vi "ClassPanel_o.vi"(8 "error in (no error)":errorcluster caption="entrée d'erreur (pas d'erreur)", 11 "AndorSpectro.lvclass":refnum<class "AndorSpectro.lvclass">) -> (0 "error out":errorcluster caption="sortie d'erreur", 3 "AndorSpectro.lvclass Out":refnum<class "AndorSpectro.lvclass">)   [LabVIEW 2019, in "AndorSpectro.lvclass"]
uses:
  AndorSpectro.lvclass
  C:/Programmes Labview/LabscanV1A/DevicesClass/BaseDevice/BaseDevice.lvclass
  <userlib>/ATSpectrograph/GUI/AndorNoiseCorr.ctl
  <userlib>/atmcd32d.llb/AndorCapabilities typedef.ctl
  <userlib>/atmcd32d.llb/TriggerMode_mode typedef.ctl
  <userlib>/atmcd32d.llb/AcquisitionMode_mode typedef.ctl
  <userlib>/atmcd32d.llb/ReadMode_mode typedef.ctl
  BaseDevice/ClassQueueMess.ctl
  AndorSpectro.lvclass/AndorSpectro.ctl
  BaseDevice/Accessor/GetClassEvent.vi
  <userlib>/ATSpectrograph/atspectrograph.lvlib
panel:
  out "Background":i32[](array[numeric])
  out "AndorMainQ":refnum<queue>
  out "Wavelength":sgl
  out "CalValues":sgl[](array[numeric])
  out "Detector offset":i32
  out "grating out":i32
  out "Grating offset":i32
  out "gain":sgl format="%.2f"
  out "information":i32
  out "caps":T1
  in  "X Start":i32=1 min=1 max=1023 step=1
  in  "X End":i32=1024 min=2 max=1024 step=1
  in  "Graph Number":i32 min=0 max=256 step=1
  in  "AndorTabs":enum32{"Main Controls", "Settings", "Data"}(tab)
  in  "AccDone":u16 caption="Acq. Done"
  in  "Stop Acq":bool
  in  "Con/Disc.":bool
  in  "Gain":i32(ring) caption="Device Name" items=["Gain  1.0(x)", "Gain  1.7(x)"]
  in  "Image Mode":bool=TRUE
  in  "AquireImage":bool caption="MiseAJour"
  out "AcqTime":sgl caption="Acq. Time (s)" format="%#.3f"
  in  "IntegTime":u32=100 caption="Integration\nTime (ms)" min=1 max=100000 step=1
  in  "Accumulation":u16=1 min=1 max=256 step=1
  out "Temp °C":i32
  in  "Cooler":bool
  in  "Save Data":bool caption="Save\nData"
  in  "Cont. Acq.":bool caption="Cont.\nAcq."
  out "Stable":bool
  in  "Setp. °C":i32=-80
  out "Aquiring":bool
  in  "Save Bckgnd":bool caption="Save as \nBckgnd"
  out "accumulate":sgl format="%.2f"
  in  "SetAreas":bool caption="MiseAJour"
  in  "Y Bins":i32=1 min=1 max=256 step=1
  out "areas":i32[][](array[numeric])=[[1], [1], [1], [1024], [256], [1], [256]]
  in  "HS":u16(ring) caption="Hor. Spd." items=["33kHz@16bit", "50kHz@16bit", "100kHz@16bit"]
  in  "VS":u16(ring)=1 caption="Vert. Spd (us)" items=["[8.25]", "16.25", "32.25", "64.25"]
  in  "Y End":i32=256 min=2 max=256 step=1
  in  "Y Start":i32=1 min=1 max=255 step=1
  in  "Backgnd Mode":T2=enum."Selected Curve"
  in  "NoiseWindow":bool caption="Noise Window"
  out "Cosmic Filter":bool
  in  "MainProgQ":refnum<queue>
  in  "MainProgQEvent":refnum<user-event>
  in  "Acq":bool
  in  "Stop":bool
  out "Init Program":bool
  # "Andor Camera"
  # "this MUST labeled with class name"
  # "this MUST be present and labeled \"Stop\" and \"Acq\""
  # "Single Acq"
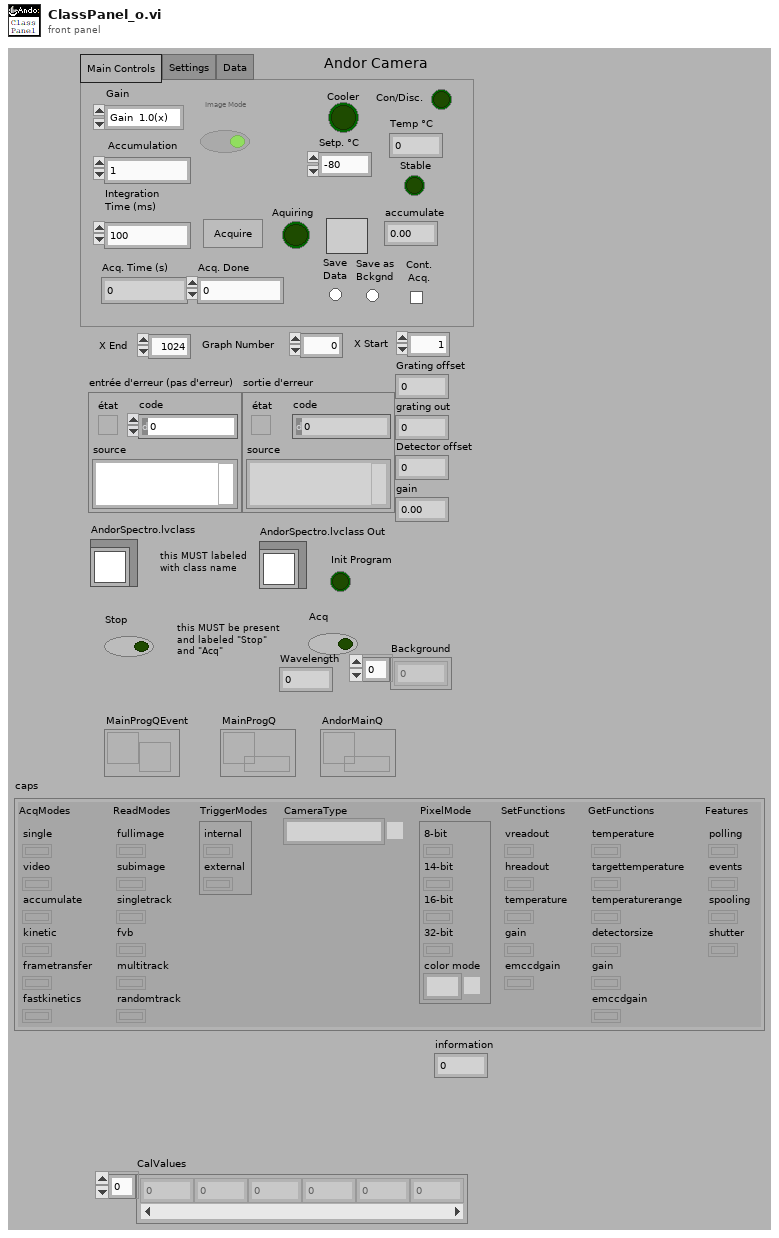
[diagram p1: front panel]
types:
  T1 = typedef "AndorCapabilities typedef.ctl" = cluster{"AcqModes":cluster{"single":bool, "video":bool, "accumulate":bool, "kinetic":bool, "frametransfer":bool, "fastkinetics":bool}, "ReadModes":cluster{"fullimage":bool, "subimage":bool, "singletrack":bool, "fvb":bool, "multitrack":bool, "randomtrack":bool}, "TriggerModes":cluster{"internal":bool, "external":bool}, "CameraType":enum32{"PDA", "iXon", "ICCD", "EMCCD", "CCD", "iStar", "third party camera", "iDus", "Newton", "Surcam", "USB ICCD", "Luca", "Reserved", "iKon", "InGaAs", "iVac", "Unprogrammed", "Clara", "USB iStar", "SimCam", "Neo", "iXon Ultra", "Volmos", "iVac Ultra"}, "PixelMode":cluster{"8-bit":bool, "14-bit":bool, "16-bit":bool, "32-bit":bool, "color mode":enum16{"Mono", "RGB", "CMY"}}, "SetFunctions":cluster{"vreadout":bool, "hreadout":bool, "temperature":bool, "gain":bool, "emccdgain":bool}, "GetFunctions":cluster{"temperature":bool, "targettemperature":bool, "temperaturerange":bool, "detectorsize":bool, "gain":bool, "emccdgain":bool}, "Features":cluster{"polling":bool, "events":bool, "spooling":bool, "shutter":bool}}
  T2 = typedef "AndorNoiseCorr.ctl" = enum16{"Off", "Selected Curve", "One For Every Acq"}
  T3 = cluster{"Message":string, "Data":variant, "Code":i32}
  T4 = typedef "ReadMode_mode typedef.ctl" = enum16{"Full Vertical Binning", "Multi-Track", "Random-Track", "Single-Track", "Image"}
  T5 = typedef "AcquisitionMode_mode typedef.ctl" = enum16{"Reserved (0)", "Single Scan", "Accumulate", "Kinetics", "Fast Kinetics", "Run Till Abort", "Reserved (6)", "Reserved (7)", "Reserved (8)", "Time Delayed Integration"}
  T6 = typedef "TriggerMode_mode typedef.ctl" = enum16{"Internal", "External", "N/A (2)", "N/A (3)", "N/A (4)", "N/A (5)", "External Start"}
  T7 = typedef "ClassQueueMess.ctl" = u16
  T8 = cluster{"wavelength out":sgl, "calibrationValuesOut":sgl[], "gain":sgl, bool}
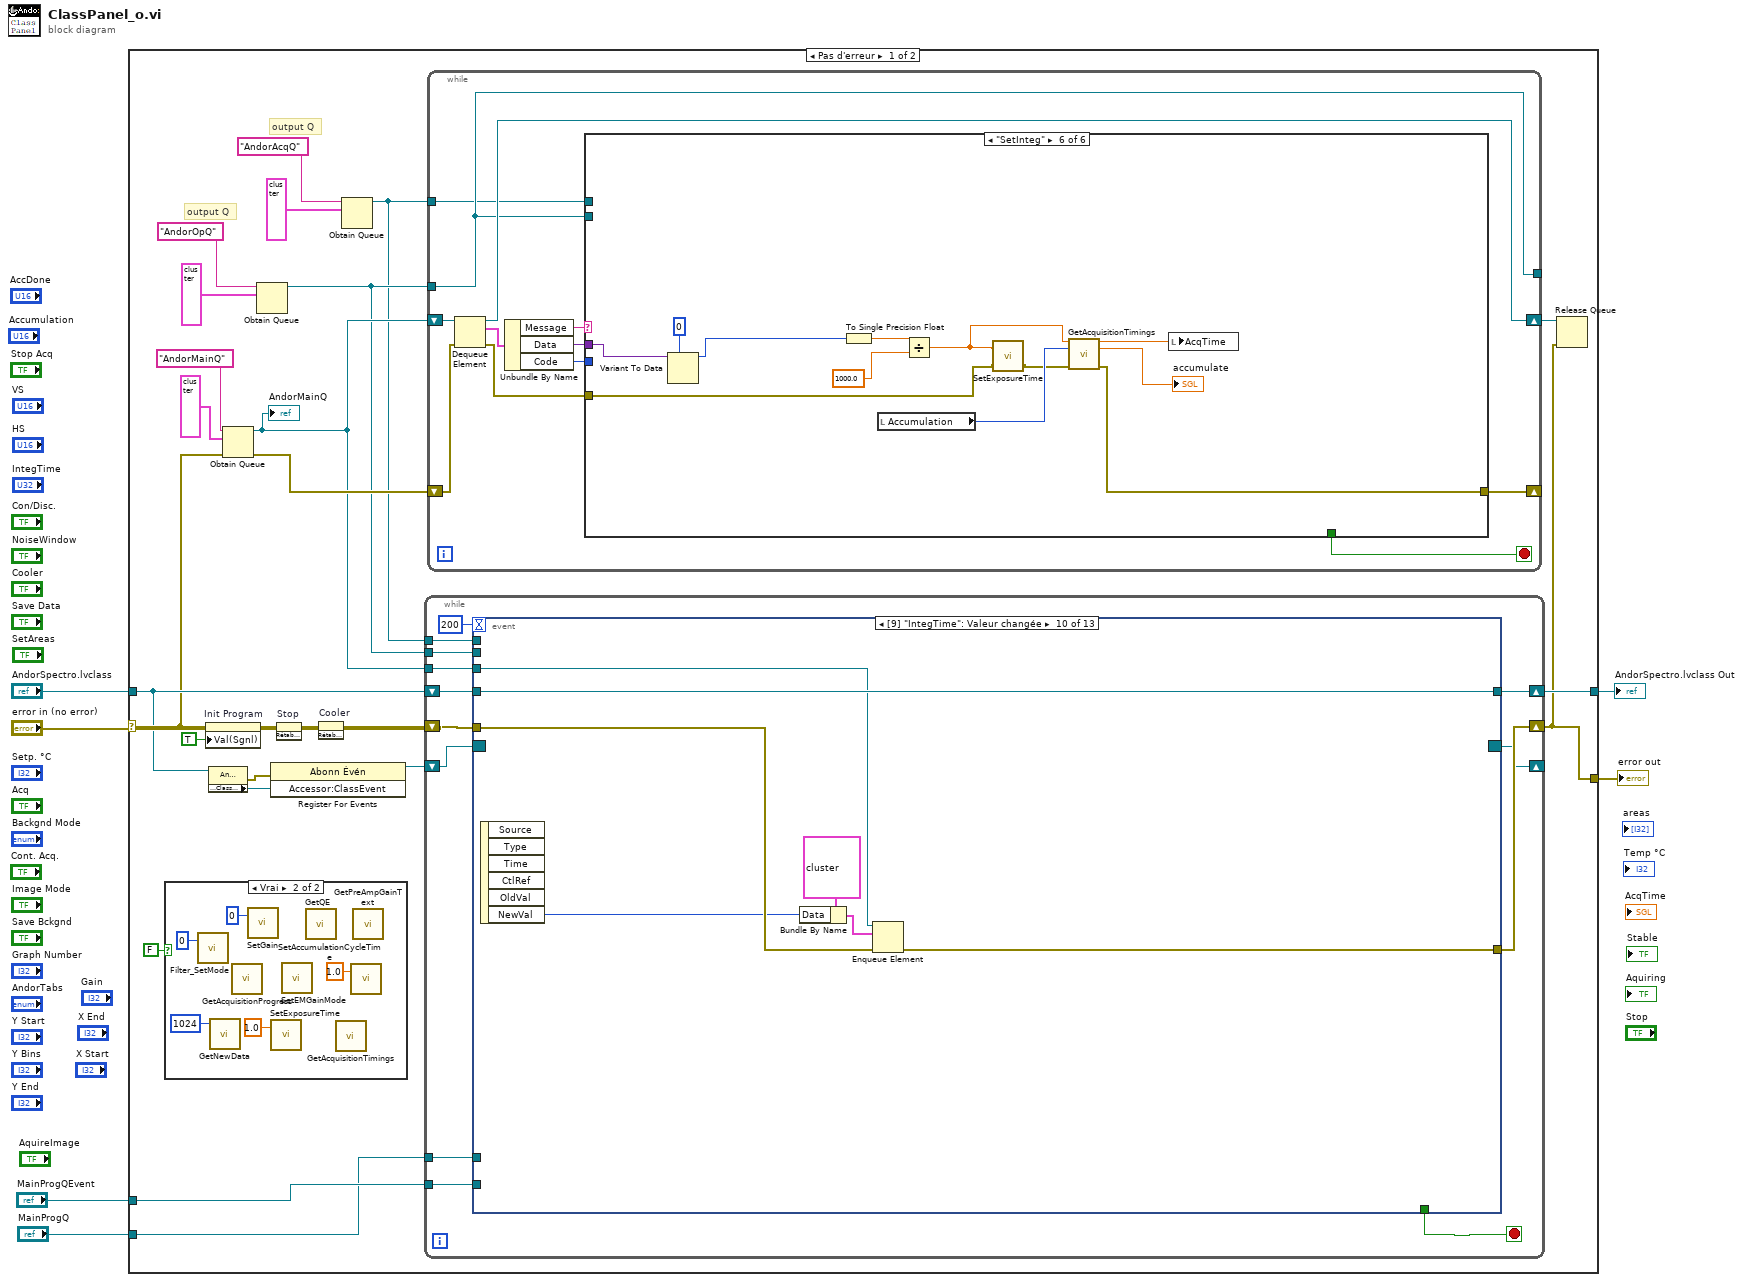
[diagram p0: block diagram]
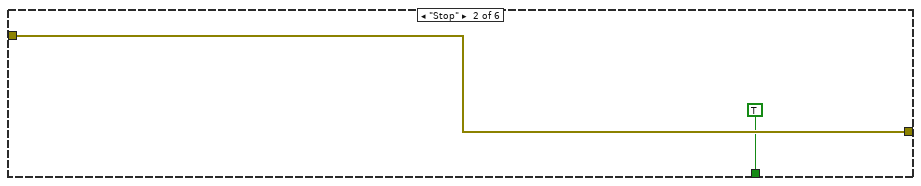
[diagram p4: hidden frame]
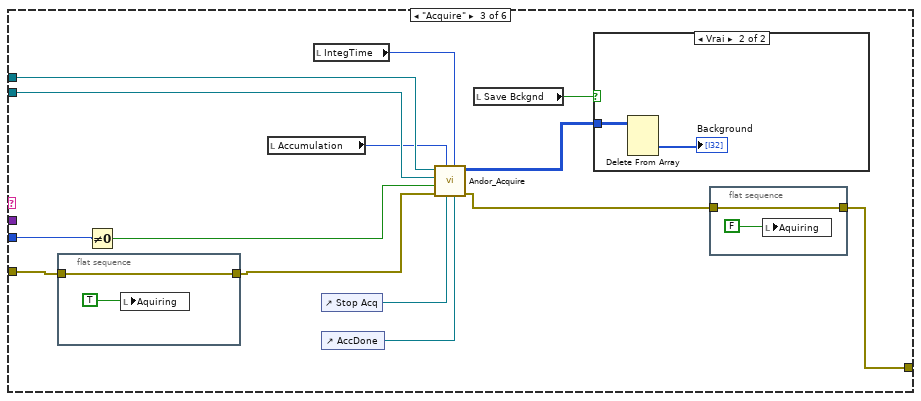
[diagram p5: hidden frame]
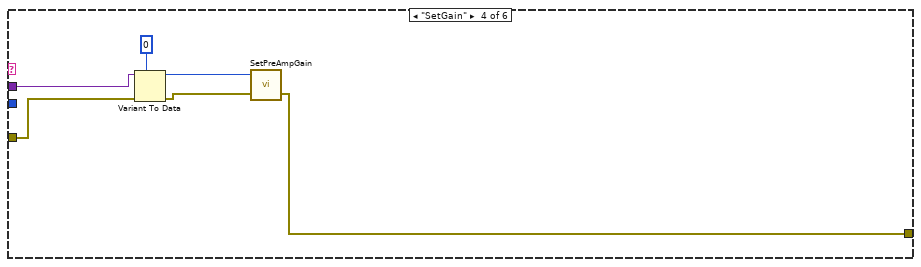
[diagram p7: hidden frame]
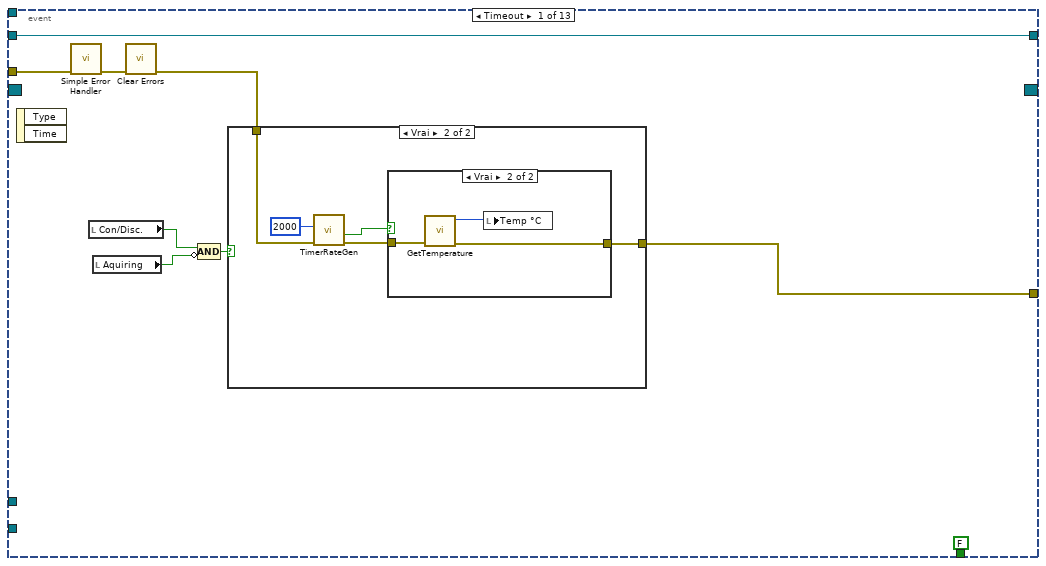
[diagram p9: hidden frame]
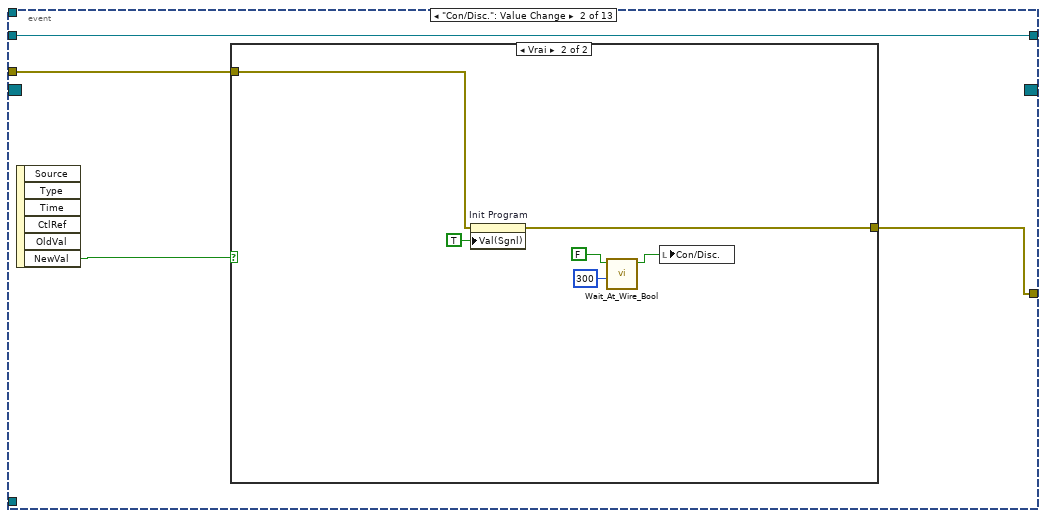
[diagram p12: hidden frame]
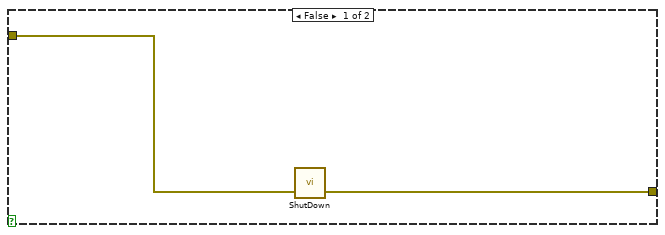
[diagram p13: hidden frame]
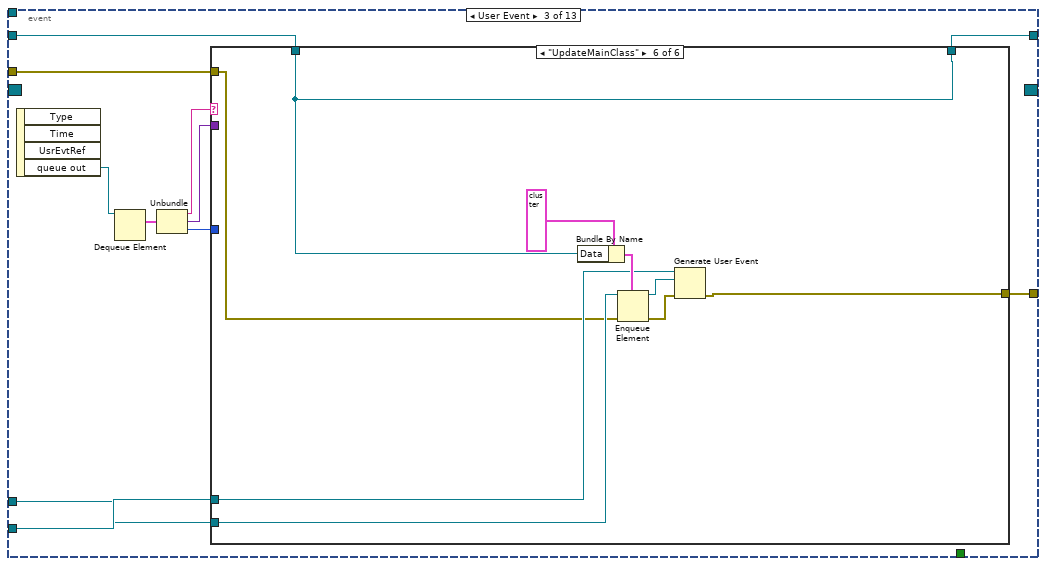
[diagram p14: hidden frame]
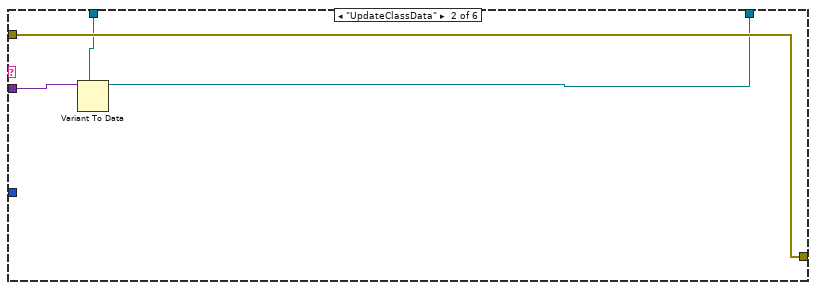
[diagram p16: hidden frame]
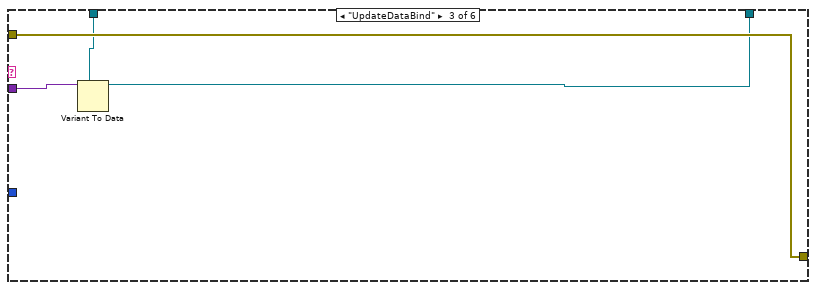
[diagram p17: hidden frame]
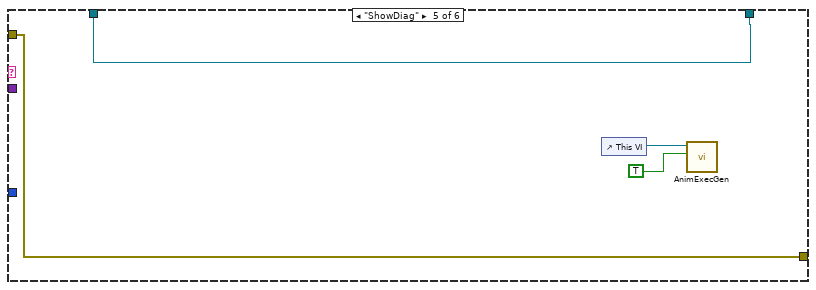
[diagram p19: hidden frame]
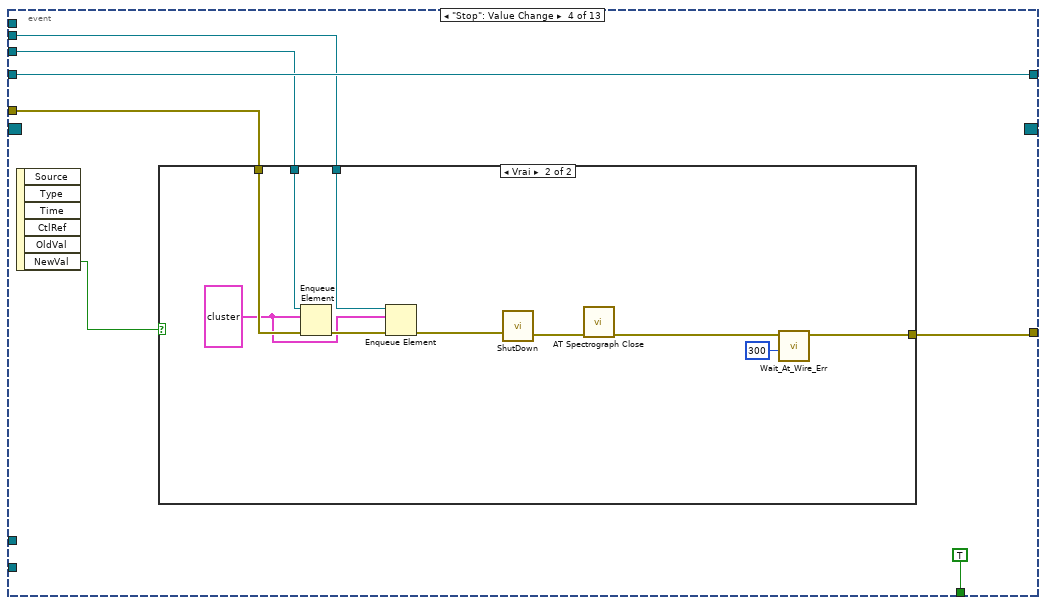
[diagram p20: hidden frame]
diagram:
  n1 = case shown="Pas d'erreur" "error in (no error)" {
    selector: "error in (no error)" -> [w21 w397]
    tunnel: [w7 w397] -> w5
    tunnel: "AndorSpectro.lvclass" -> [w26 w396]
    tunnel: [w30 w396] -> w3
    tunnel: "MainProgQEvent" -> [w24 _]
    tunnel: "MainProgQ" -> [w23 _]
    frame No Error {
      # "output Q"
      # "output Q"
      n2 = case shown="Vrai" FALSE {
        frame False {
        }
        frame True {
          n3 = call <userlib>:"Filter_SetMode.vi"("Mode"=u32 0) -> ()  [unwired: 1 in, 2 out]
          n4 = call <userlib>:"GetNewData.vi"("size"=u32 1024) -> ()  [unwired: 2 in, 3 out]
          n5 = call <userlib>:"GetAcquisitionProgress.vi"() -> ()  [unwired: 4 in, 4 out]
          n6 = call <userlib>:"SetGain.vi"("gain"=0) -> ()  [unwired: 1 in, 2 out]
          n7 = call <userlib>:"SetExposureTime.vi"("time"=sgl 1.0) -> ()  [unwired: 1 in, 2 out]
          n8 = call <userlib>:"SetEMGainMode.vi"() -> ()  [unwired: 2 in, 2 out]
          n9 = call <userlib>:"GetQE.vi"() -> ()  [unwired: 4 in, 3 out]
          n10 = call <userlib>:"GetAcquisitionTimings.vi"() -> ()  [unwired: 11 in, 5 out]
          n11 = call <userlib>:"SetAccumulationCycleTime.vi"("time"=sgl 1.0) -> ()  [unwired: 1 in, 2 out]
          n12 = call <userlib>:"GetPreAmpGainText.vi"() -> ()  [unwired: 2 in, 3 out]
        }
      }
      n13 = property on="Init Program" class="Bool (strict)"(error in=w21, "Val(Sgnl)"=TRUE ("Valeur (Signalisation)")) -> (error out=w29:errorcluster)  [unwired: 1 in, 1 out]
      n14 = property class="AndorSpectro.lvclass"(reference=w26) -> (error out=w28:errorcluster, "Accessor:ClassEvent"=w27:refnum<user-event>)  [unwired: 1 in, 1 out]
      n15 = Obtain Queue(name (unnamed)="AndorMainQ" ("nom (aucun)"), element data type=T3 {"Message"="", "Data"=variant, "Code"=0}, error in (no error)=w21) -> (queue out=w18:refnum<queue>, error out=w20:errorcluster)  [unwired: 2 in, 1 out]
      "AndorMainQ" <- w18
      n16 = Obtain Queue(name (unnamed)="AndorOpQ" ("nom (aucun)"), element data type=T3 {"Message"="", "Data"=variant, "Code"=0} ("element")) -> (queue out=w11:refnum<queue>)  [unwired: 3 in, 2 out]
      n17 = register-events(error in=w28, w27) -> (reference out=w25:refnum<event-registration>)  [unwired: 1 in, 1 out]
      n18 = invoke on="Stop" class="Bool (strict)" method="RétablirValParDéfaut"(error in=w29) -> (error out=w13:errorcluster)  [unwired: 2 in, 2 out]
      n19 = invoke on="Cooler" class="Bool (strict)" method="RétablirValParDéfaut"(error in=w13) -> (error out=w12:errorcluster)  [unwired: 2 in, 2 out]
      n20 = Obtain Queue(name (unnamed)="AndorAcqQ" ("nom (aucun)"), element data type=T3 {"Message"="", "Data"=variant, "Code"=0} ("element")) -> (queue out=w8:refnum<queue>)  [unwired: 3 in, 2 out]
      n21 = while {
        shift-right: [w101] -> w7
        shift-left: w12 -> [w102]
        shift-right: [w99] -> w30
        shift-left: w26 -> [w100]
        shift-right: [w97] -> _
        shift-left: w25 -> [w98]
        tunnel: w24 -> [w96]
        tunnel: w23 -> [w95]
        tunnel: w18 -> [w94]
        tunnel: w11 -> [w93]
        tunnel: w8 -> [w92]
        stop <- w91 stop-if-true
        n22 = event shown="[9] \"IntegTime\": Valeur changée" {
          selector: w98 -> [_ _ _ _ _ _ _ _ _ _ _ _ _]
          dyn-events: [_ _ _ _ _ _ _ _ _ _ _ _ _] -> w97
          timeout: 200 -> [_ _ _ _ _ _ _ _ _ _ _ _ _]
          tunnel: w102 -> [w110 w125 w144 w174 w189 w197 w293 w305 w315 w325 w335 w372 w391]
          tunnel: [w106 w123 w138 w172 w189 w199 w289 w304 w314 w327 w331 w371 w390] -> w101
          tunnel: w100 -> [w111 w124 w145 w176 w190 w194 w294 w306 w317 w328 w336 w373 w395]
          tunnel: [FALSE _ _ TRUE _ FALSE _ _ _ _ _ _ _] -> w91
          tunnel: [w111 w124 w137 w176 w190 w193 w294 w306 w317 w328 w332 w373 w395] -> w99
          tunnel: w96 -> [_ _ w136 _ _ _ _ _ _ _ w333 _ _]
          tunnel: w95 -> [_ _ w135 _ _ _ _ _ _ _ w334 _ _]
          tunnel: w94 -> [_ _ _ w175 _ w195 w288 _ _ w326 w330 _ w389]
          tunnel: w93 -> [_ _ _ w173 _ w196 _ _ _ _ w329 _ _]
          tunnel: w92 -> [_ _ _ _ _ w192 _ _ _ _ _ _ _]
          event Timeout {
            n23 = event-data() -> ()  [unwired: 1 in, 2 out]
            n24 = call <vilib>:"Simple Error Handler.vi"("error in (no error)"=w110) -> ("error out"=w109:errorcluster)  [unwired: 4 in, 4 out]
            n25 = local read "Con/Disc."() -> (w108:bool)
            n26 = local read "Aquiring"() -> (w104:bool)
            n27 = call <vilib>:"Clear Errors.vi"("error in (no error)"=w109) -> ("error out"=w107:errorcluster)  [unwired: 5 in, 1 out]
            n28 = Compound Arithmetic op=AND ("Opérateur arithmétique")(w108, invert w104) -> (w105:bool)
            n29 = case shown="Vrai" w105 {
              tunnel: w107 -> [w113 w117]
              tunnel: [w113 w115] -> w106
              frame False {
              }
              frame True {
                n30 = call <userlib>:"TimerRateGen.vi"("error in (no error)"=w117, "Refresh(ms)"=u32 2000) -> ("error out"=w116:errorcluster, "updated?"=w114:bool)  [unwired: 7 in, 1 out]
                n31 = case shown="Vrai" w114 {
                  tunnel: w116 -> [w119 w122]
                  tunnel: [w119 w120] -> w115
                  frame False {
                  }
                  frame True {
                    n32 = call <userlib>:"GetTemperature.vi"("error in (no error)"=w122) -> ("error out"=w120:errorcluster, "temperature"=w121:i32)  [unwired: 3 in, 2 out]
                    n33 = local write "Temp °C"(w121) -> ()
                  }
                }
              }
            }
          }
          event "Con/Disc.": Value Change {
            n34 = event-data() -> ("NewVal"=w126:bool)  [unwired: 1 in, 5 out]
            n35 = case shown="Vrai" w126 {
              tunnel: w125 -> [w128 w133]
              tunnel: [w127 w132] -> w123
              frame False {
                n36 = call <userlib>:"ShutDown.vi"("error in (no error)"=w128) -> ("error out"=w127:errorcluster)  [unwired: 1 in, 1 out]
              }
              frame True {
                n37 = property on="Init Program" class="Bool (strict)"(error in=w133, "Val(Sgnl)"=TRUE ("Valeur (Signalisation)")) -> (error out=w132:errorcluster)  [unwired: 1 in, 1 out]
                n38 = call <userlib>:"Wait_At_Wire_Bool.vi"("Wait (ms)"=u32 300, "error in (no error)"=FALSE ("Con/Disc.")) -> ("error out"=w130:bool)  [unwired: 7 in, 2 out]
                n39 = local write "Con/Disc."(w130) -> ()
              }
            }
          }
          event User Event {
            n40 = event-data() -> ("queue out"=w142:refnum<queue>)  [unwired: 1 in, 3 out]
            n41 = Dequeue Element(queue=w142) -> (element=w143:cluster{"Message":string, "Data":variant, i32})  [unwired: 2 in, 3 out]
            n42 = Unbundle(w143) -> ("Message"=w141:string, "Data"=w140:variant, w139:i32)
            n43 = case shown="\"UpdateMainClass\"" w141 {
              tunnel: w144 -> [w147 w151 w155 w156 w160 w163]
              tunnel: w140 -> [_ w150 w154 _ _ _]
              tunnel: w145 -> [w146 w149 w153 w157 w161 w166]
              tunnel: [w146 w148 w152 w157 w161 w166] -> w137
              tunnel: [w147 w151 w155 w156 w160 w162] -> w138
              tunnel: w139 -> [_ _ _ _ _ _]
              tunnel: w136 -> [_ _ _ _ _ w165]
              tunnel: w135 -> [_ _ _ _ _ w164]
              frame Default {
              }
              frame "UpdateClassData" {
                n44 = Variant To Data(type=w149, Variant=w150) -> (data=w148:refnum<class "AndorSpectro.lvclass">)  [unwired: 1 in, 1 out]
              }
              frame "UpdateDataBind" {
                n45 = Variant To Data(type=w153, Variant=w154) -> (data=w152:refnum<class "AndorSpectro.lvclass">)  [unwired: 1 in, 1 out]
              }
              frame "MeasDone" {
              }
              frame "ShowDiag" {
                n46 = control-ref of="This VI"() -> (w159:refnum<vi>)
                n47 = call <userlib>:"AnimExecGen.vi"("Animer l'exécution ?"=TRUE, "ViRef"=w159) -> ()  [unwired: 9 in, 1 out]
              }
              frame "UpdateMainClass" {
                n48 = Bundle By Name(cluster=cluster{"Message":string, "Data":variant, i32} {"Message"="", "Data"=variant, 0} ("élément"), "Data"=w166) -> (w167:cluster{"Message":string, "Data":variant, i32})
                n49 = Enqueue Element(queue=w164, element=w167, error in (no error)=w163) -> (queue out=w170:refnum<queue>, error out=w169:errorcluster)  [unwired: 1 in, 1 out]
                n50 = Generate User Event(user event=w165, event data cluster=w170, error in=w169) -> (error out=w162:errorcluster)  [unwired: 1 in, 1 out]
              }
            }
          }
          event "Stop": Value Change {
            n51 = event-data() -> ("NewVal"=w171:bool)  [unwired: 1 in, 5 out]
            n52 = case shown="Vrai" w171 {
              tunnel: w175 -> [_ w188]
              tunnel: w174 -> [w178 w187]
              tunnel: w173 -> [_ w183]
              tunnel: [w178 w180] -> w172
              frame False {
              }
              frame True {
                w182 = T3 {"Message"="Stop", "Data"=variant, "Code"=0} ("élément")
                n53 = Enqueue Element(queue=w188, element=w182, error in (no error)=w187) -> (error out=w184:errorcluster)  [unwired: 1 in, 2 out]
                n54 = Enqueue Element(queue=w183, element=w182, error in (no error)=w184) -> (error out=w181:errorcluster)  [unwired: 1 in, 2 out]
                n55 = call <userlib>:"ShutDown.vi"("error in (no error)"=w181) -> ("error out"=w186:errorcluster)  [unwired: 1 in, 1 out]
                n56 = call <userlib>:"AT Spectrograph Close.vi"("error in (no error)"=w186) -> ("error out"=w185:errorcluster)  [unwired: 9 in, 1 out]
                n57 = call <userlib>:"Wait_At_Wire_Err.vi"("Wait (ms)"=u32 300, "error in (no error)"=w185) -> ("error out"=w180:errorcluster)  [unwired: 7 in, 2 out]
              }
            }
          }
          event Panel Close? {
            n58 = event-data() -> ()  [unwired: 1 in, 4 out]
            n59 = event-data("Discard?"=TRUE ("Rejeter ?")) -> ()  [unwired: 1 in, 1 out]
          }
          event "Init Program": Value Change {
            n60 = event-data() -> ("NewVal"=w200:bool)  [unwired: 1 in, 4 out]
            n61 = case shown="Vrai" w200 {
              tunnel: w197 -> [w202 w204]
              tunnel: [w202 w222] -> w199
              tunnel: [_ w240] -> _
              tunnel: [_ w239] -> _
              tunnel: [_ w235] -> _
              tunnel: [_ w221] -> _
              tunnel: w196 -> [_ w215]
              tunnel: w195 -> [_ w209]
              tunnel: w194 -> [w201 w216]
              tunnel: [w201 w211] -> w193
              tunnel: w192 -> [_ w210]
              frame False {
              }
              frame True {
                w213 = T7 1 items=["UpdateClassData", "UpdateMainClass", "UpdateDataBind", "ReInitDevice", "Custom", "ClosePan"] ("Menu déroulant")
                w245 = u32 0 items=["DIRECT", "SIDE"] ("entrancePort")
                w246 = u32 0 items=["DIRECT", "SIDE"] ("exitPort")
                w229 = 0
                w231 = 0
                w254 = 0 ("index")
                w274 = -80 ("temperature")
                w271 = 0
                w283 = u32 20002  # DRV_SUCCESS
                n62 = call <userlib>:"Initialize.vi"("error in (no error)"=w204, "directory (\"\")"="" ("directory (\"\")")) -> ("error out"=w264:errorcluster, "DLL error code"=w284:u32)
                n63 = local write "Image Mode"(FALSE ("Image Mode")) -> ()
                n64 = call <userlib>:"Wait_At_Wire_Err.vi"("Wait (ms)"=u32 2000, "error in (no error)"=w264) -> ("error out"=w262:errorcluster)  [unwired: 7 in, 2 out]
                n65 = Equal?(x=w284, y=w283) -> (x = y?=w260:bool)
                n66 = Open VI Reference(type specifier VI Refnum (for type only)=refnum<vi> refnum ("référence"), vi path=path "C:/Program Files (x86)/National Instruments/LabVIEW 2019/user.lib/ATSpectrograph/GUI/Andor_Operate.vi" ("chemin du VI"), options=128, error in (no error)=w204) -> (vi reference=w205:refnum<vi>, error out=w203:errorcluster)  [unwired: 2 in]
                n67 = call <userlib>:"GetCameraInformation.vi"("error in (no error)"=w262) -> ("error out"=w263:errorcluster, "information"=w259:i32)  [unwired: 2 in, 1 out]
                "information" <- w259
                n68 = Equal?(x=7, y=w259) -> (x = y?=w257:bool)
                n69 = call-by-ref "Démarrer un appel asynchrone"(reference=w205, error in=w203, 8:"error in (no error)"=w204, "AndorAcqQ"=w209, "AndorOpQ"=w215) -> ()  [unwired: 8 in, 3 out]
                n70 = call <userlib>:"GetCapabilities.vi"("error in (no error)"=w263) -> ("error out"=w261:errorcluster, "caps"=→"caps":T1)  [unwired: 2 in, 1 out]
                n71 = And(x=w260, y=w257) -> (x .and. y?=w217:bool)
                n72 = local write "Con/Disc."(w217) -> ()
                n73 = property on="Accumulation" class="NumNb (strict)"("Value"=u16 1 ("Accumulation")) -> ()  [unwired: 2 in, 2 out]
                n74 = call <userlib>:"SetReadMode.vi"("error in (no error)"=w261, "mode"=ReadMode_mode_typedef."Full Vertical Binning") -> ("error out"=w280:errorcluster)  [unwired: 1 out]
                n75 = call <userlib>:"SetAcquisitionMode.vi"("error in (no error)"=w280, "mode"=AcquisitionMode_mode_typedef."Single Scan") -> ("error out"=w253:errorcluster)  [unwired: 1 out]
                n76 = local write "Setp. °C"(w274) -> ()
                n77 = Bundle By Name(cluster=w216, "AndorOpQ"=w215, "AndorAcqQ"=w210, "AndorMainQ"=w209) -> (w214:refnum<class "AndorSpectro.lvclass">)
                n78 = call <userlib>:"GetPreAmpGain.vi"("error in (no error)"=w253, "index"=w254) -> ("gain"=w218:sgl)  [unwired: 1 in, 2 out]
                "gain" <- w218
                n79 = call <userlib>:"SetPreAmpGain.vi"("error in (no error)"=w253, "index"=w254) -> ("error out"=w268:errorcluster)  [unwired: 1 out]
                n80 = property on="Gain" class="MDér (strict)"(error in=w253, "Value"=w254) -> (error out=w267:errorcluster)  [unwired: 1 in, 1 out]
                n81 = call <userlib>:"SetHSSpeed.vi"("error in (no error)"=w268, "index"=w271, "type"=w271) -> ("error out"=w277:errorcluster)  [unwired: 1 in, 1 out]
                n82 = property on="HS" class="MDér (strict)"(error in=w267, "Value"=w271) -> (error out=w266:errorcluster)  [unwired: 1 in, 1 out]
                n83 = call <userlib>:"GetNumberVSSpeeds.vi"("error in (no error)"=w277) -> ("error out"=w276:errorcluster, "number"=w278:i32)  [unwired: 2 in, 1 out]
                n84 = Subtract(x=w278, y=1) -> (x-y=w272:i32)
                n85 = call <userlib>:"SetVSSpeed.vi"("error in (no error)"=w276, "index"=w272) -> ("error out"=w241:errorcluster)  [unwired: 1 out]
                n86 = property on="VS" class="MDér (strict)"(error in=w266, "Value"=w272) -> (error out=w212:errorcluster)  [unwired: 1 in, 1 out]
                n87 = call <userlib>:"GetPixelSize.vi"("error in (no error)"=w241) -> ("error out"=w242:errorcluster, "ysize"=w239:sgl, "xsize"=w240:sgl)  [unwired: 3 in, 1 out]
                n88 = call-dynamic "SetClassQueueMessage.vi"("ErrorIn(No Error)"=w212, "Menu déroulant"=w213, "DefaultDev.lvclass"=w214) -> ("DefaultDev.lvclass Out"=w211:refnum<class "AndorSpectro.lvclass">)  [unwired: 7 in, 1 out]
                n89 = call <userlib>:"GetFilterMode.vi"("error in (no error)"=w242) -> ("error out"=w238:errorcluster, "mode"=→"Cosmic Filter":bool)  [unwired: 2 in, 1 out]
                n90 = call <userlib>:"SetTemperature.vi"("error in (no error)"=w238, "temperature"=w274) -> ("error out"=w273:errorcluster)  [unwired: 1 out]
                n91 = call <userlib>:"SetTriggerMode.vi"("error in (no error)"=w273, "mode"=TriggerMode_mode_typedef."Internal") -> ("error out"=w234:errorcluster)  [unwired: 1 out]
                n92 = property on="IntegTime" class="NumNb (strict)"(error in=w234, "Val(Sgnl)"=u32 100 ("Valeur (Signalisation)")) -> (error out=w237:errorcluster)  [unwired: 1 in, 1 out]
                n93 = call <userlib>:"AT Spectrograph Initialize.vi"("error in (no error)"=w237, "iniPath"="") -> ("error out"=w233:errorcluster, "function return"=w235:u32)  [unwired: 8 in]
                n94 = call <userlib>:"AT Spectrograph Get Wavelength.vi"("error in (no error)"=w233, "device"=w231) -> ("error out"=w232:errorcluster, "wavelength out"=w221:sgl)  [unwired: 7 in, 1 out]
                "Wavelength" <- w221
                n95 = call <userlib>:"AT Spectrograph Set Pixel Width.vi"("error in (no error)"=w232, "width"=sgl 26.0, "device"=w231) -> ("error out"=w251:errorcluster)  [unwired: 7 in, 1 out]
                n96 = call <userlib>:"AT Spectrograph Set Number Pixels.vi"("error in (no error)"=w251, "numberPixels"=1024, "device"=w231) -> ("error out"=w227:errorcluster)  [unwired: 7 in, 1 out]
                n97 = call <userlib>:"AT Spectrograph Get Grating.vi"("error in (no error)"=w227, "device"=w229) -> ("error out"=w226:errorcluster, "grating out"=w247:i32)  [unwired: 7 in, 1 out]
                "grating out" <- w247
                n98 = call <userlib>:"AT Spectrograph Get Grating Offset.vi"("error in (no error)"=w226, "grating"=w247, "device"=w229) -> ("error out"=w249:errorcluster, "offset out"=→"Grating offset":i32)  [unwired: 6 in, 1 out]
                n99 = call <userlib>:"AT Spectrograph Get Detector Offset.vi"("error in (no error)"=w249, "exitPort"=w246, "entrancePort"=w245, "device"=w229) -> ("error out"=w228:errorcluster, "offset out"=→"Detector offset":i32)  [unwired: 5 in, 1 out]
                n100 = call <userlib>:"AT Spectrograph Get Calibration.vi"("error in (no error)"=w228, "numberPixels"=1024, "device"=w229) -> ("error out"=w223:errorcluster, "calibrationValuesOut"=w220:sgl[])  [unwired: 5 in, 1 out]
                "CalValues" <- w220
                n101 = Bundle("wavelength out"=w221, "calibrationValuesOut"=w220, "gain"=w218, w217) -> (w219:T8)  [unwired: 1 in]
                n102 = Bundle By Name(cluster=T3 {"Message"="InitOp", "Data"=variant, "Code"=1}, "Data"=w219) -> (w225:T3)
                n103 = Enqueue Element(queue=w215, element=w225, error in (no error)=w223) -> (error out=w222:errorcluster)  [unwired: 1 in, 2 out]
                "Init Program" <- FALSE
              }
            }
          }
          event "Accumulation": Value Change {
            n104 = event-data() -> ("NewVal"=w295:u16)  [unwired: 1 in, 5 out]
            n105 = case shown="1" w295 {
              selector: w295 -> [w296 _]
              tunnel: w293 -> [w300 w303]
              tunnel: [w297 w302] -> w290
              frame Default {
                n106 = call <userlib>:"SetAcquisitionMode.vi"("error in (no error)"=w300, "mode"=AcquisitionMode_mode_typedef."Accumulate") -> ("error out"=w298:errorcluster)  [unwired: 1 out]
                n107 = call <userlib>:"SetNumberAccumulations.vi"("error in (no error)"=w298, "number"=w296) -> ("error out"=w297:errorcluster)  [unwired: 1 out]
              }
              frame 1 {
                # "Single scan mode"
                n108 = call <userlib>:"SetAcquisitionMode.vi"("error in (no error)"=w303, "mode"=AcquisitionMode_mode_typedef."Single Scan") -> ("error out"=w302:errorcluster)  [unwired: 1 out]
              }
            }
            n109 = local read "IntegTime"() -> (w287:u32)
            n110 = Bundle By Name(cluster=T3 {"Message"="SetInteg", "Data"=variant, "Code"=0}, "Data"=w287) -> (w291:T3)
            n111 = Enqueue Element(queue=w288, element=w291, error in (no error)=w290) -> (error out=w289:errorcluster)  [unwired: 1 in, 2 out]
          }
          event "Cont. Acq.": Value Change {
            n112 = event-data() -> ("NewVal"=w307:bool)  [unwired: 1 in, 5 out]
            n113 = case shown="Faux" w307 {
              tunnel: w305 -> [w310 w312]
              tunnel: [w309 w311] -> w304
              frame False {
                n114 = local read "Accumulation"() -> (w308:u16)
                n115 = property on="Accumulation" class="NumNb (strict)"(error in=w310, "Val(Sgnl)"=w308) -> (error out=w309:errorcluster)  [unwired: 1 in, 1 out]
              }
              frame True {
                n116 = call <userlib>:"SetAcquisitionMode.vi"("error in (no error)"=w312, "mode"=AcquisitionMode_mode_typedef."Run Till Abort") -> ("error out"=w311:errorcluster)  [unwired: 1 out]
              }
            }
          }
          event "Cooler": Value Change {
            n117 = event-data() -> ("NewVal"=w316:bool)  [unwired: 1 in, 5 out]
            n118 = case shown="Faux" w316 {
              tunnel: w315 -> [w319 w321]
              tunnel: [w318 w320] -> w314
              frame False {
                n119 = call <userlib>:"CoolerOFF.vi"("error in (no error)"=w319) -> ("error out"=w318:errorcluster)  [unwired: 1 in, 1 out]
              }
              frame True {
                n120 = call <userlib>:"CoolerON.vi"("error in (no error)"=w321) -> ("error out"=w320:errorcluster)  [unwired: 1 in, 1 out]
              }
            }
          }
          event "IntegTime": Value Change {
            n121 = event-data() -> ("NewVal"=w322:u32)  [unwired: 1 in, 5 out]
            n122 = Bundle By Name(cluster=T3 {"Message"="SetInteg", "Data"=variant, "Code"=0}, "Data"=w322) -> (w323:T3)
            n123 = Enqueue Element(queue=w326, element=w323, error in (no error)=w325) -> (error out=w327:errorcluster)  [unwired: 1 in, 2 out]
          }
          event "AquireImage": Value Change {
            n124 = event-data() -> ("NewVal"=w337:bool)  [unwired: 1 in]
            n125 = case shown="Vrai" w337 {
              tunnel: w336 -> [w338 w351]
              tunnel: w335 -> [w339 w342]
              tunnel: w334 -> [_ w349]
              tunnel: w333 -> [_ w350]
              tunnel: [w338 w348] -> w332
              tunnel: [w339 w346] -> w331
              tunnel: w330 -> [_ w340]
              tunnel: w329 -> [_ _]
              frame False {
              }
              frame True {
                n126 = local read "Save Data"() -> (w341:bool)
                n127 = property class="AndorSpectro.lvclass"(reference=w351, error in=w342) -> (reference out=w348:refnum<class "AndorSpectro.lvclass">, error out=w347:errorcluster, "Accessor:Function"=w356:string, "Accessor:InstrumentName"=w354:string)
                n128 = Concatenate Strings(w356, "@" ("chaîne"), w354) -> (w352:string)
                n129 = Bundle(w352, "Save Data"=w341) -> (w353:cluster{string, "Save Data":bool})  [unwired: 1 in]
                n130 = case shown="Faux" w341 {
                  tunnel: w353 -> [_ w365]
                  tunnel: w350 -> [_ w364]
                  tunnel: w349 -> [_ w363]
                  tunnel: w347 -> [w359 w362]
                  tunnel: [w358 w361] -> w346
                  tunnel: w340 -> [w360 _]
                  frame False {
                    n131 = Enqueue Element(queue=w360, element=T3 {"Message"="Acquire", "Data"=variant, "Code"=0}, error in (no error)=w359) -> (error out=w358:errorcluster)  [unwired: 1 in, 2 out]
                  }
                  frame True {
                    n132 = To Variant(anything=w365) -> (Variant=w368:variant)
                    n133 = Bundle By Name(cluster=cluster{"Message":string, "Data":variant, i32} {"Message"="ArrayDevAcqSetup", "Data"=variant, 0} ("élément"), "Data"=w368) -> (w367:cluster{"Message":string, "Data":variant, i32})
                    n134 = Enqueue Element(queue=w363, element=w367, error in (no error)=w362) -> (queue out=w370:refnum<queue>, error out=w366:errorcluster)  [unwired: 1 in, 1 out]
                    n135 = Generate User Event(user event=w364, event data cluster=w370, error in=w366) -> (error out=w361:errorcluster)  [unwired: 1 in, 1 out]
                  }
                }
                n136 = call <userlib>:"Wait_At_Wire_Bool.vi"("Wait (ms)"=u32 300, "error in (no error)"=FALSE) -> ("error out"=w344:bool)  [unwired: 7 in, 2 out]
                n137 = local write "AquireImage"(w344) -> ()
              }
            }
          }
          event "SetAreas": Value Change {
            n138 = event-data() -> ()  [unwired: 1 in, 6 out]
            n139 = local read "Y Start"() -> (w376:i32)
            n140 = local read "Y Bins"() -> (w378:i32)
            n141 = local read "Y End"() -> (w375:i32)
            n142 = Greater?(x=w378, y=1) -> (0:w374:bool)
            n143 = case shown="Vrai" w374 {
              tunnel: w376 -> [_ w387]
              tunnel: w375 -> [_ w388]
              tunnel: w372 -> [w379 w381]
              tunnel: [w379 w380] -> w371
              frame False {
              }
              frame True {
                n144 = Subtract(x=w388, y=w387) -> (x-y=w386:i32)
                n145 = Increment(x=w386) -> (x+1=w384:i32)
                n146 = Quotient & Remainder(x=w384, y=2) -> (floor(x/y)=w383:i32)  [unwired: 1 out]
                n147 = Increment(x=w383) -> (x+1=w382:i32)
                n148 = call <userlib>:"SetSingleTrack.vi"("error in (no error)"=w381, "height"=w384, "centre"=w382) -> ("error out"=w380:errorcluster)  [unwired: 1 in, 1 out]
              }
            }
          }
          event "Gain": Value Change {
            n149 = event-data() -> ("NewVal"=w392:i32)  [unwired: 1 in]
            n150 = Bundle By Name(cluster=cluster{"Message":string, "Data":variant, i32} {"Message"="SetGain", "Data"=variant, 0} ("ClassQueue"), "Data"=w392) -> (w393:cluster{"Message":string, "Data":variant, i32})
            n151 = Enqueue Element(queue=w389, element=w393, error in (no error)=w391) -> (error out=w390:errorcluster)  [unwired: 1 in, 2 out]
          }
        }
      }
      n152 = while {
        shift-right: [w47] -> w15
        shift-left: w18 -> [w48]
        shift-right: [w44] -> _
        shift-left: w20 -> [w42]
        tunnel: w11 -> [w39]
        tunnel: [w39] -> _
        tunnel: w8 -> [w38]
        stop <- w41 stop-if-true
        n153 = Dequeue Element(queue=w48, error in (no error)=w42) -> (queue out=w47:refnum<queue>, element=w46:T3, error out=w43:errorcluster)  [unwired: 1 in, 1 out]
        n154 = Unbundle By Name(w46) -> ("Message"=w45:string, "Data"=w40:variant, "Code"=w37:i32)
        n155 = case shown="\"SetInteg\"" w45 {
          tunnel: [w49 w51 w58 w72 w78 w84] -> w44
          tunnel: w43 -> [w49 w51 w56 w74 w78 w81]
          tunnel: [_ TRUE _ _ _ _] -> w41
          tunnel: w40 -> [_ _ _ w77 _ w86]
          tunnel: w39 -> [_ _ w65 _ _ _]
          tunnel: w38 -> [_ _ w64 _ _ _]
          tunnel: w37 -> [_ _ w63 _ _ _]
          frame "Error", Default {
          }
          frame "Stop" {
          }
          frame "Acquire" {
            n156 = flat-sequence {
              tunnel: [w68] -> w55
              tunnel: w56 -> [w68]
              frame #0 {
                n157 = local write "Aquiring"(TRUE) -> ()
              }
            }
            n158 = Not Equal To 0?(x=w63) -> (x != 0?=w62:bool)
            n159 = local read "Accumulation"() -> (w59:u16)
            n160 = local read "IntegTime"() -> (w60:u32)
            n161 = control-ref of="Stop Acq"() -> (w61:refnum<vi>)
            n162 = control-ref of="AccDone"() -> (w52:refnum<vi>)
            n163 = call <userlib>:"Andor_Acquire.vi"("AccDoneRef"=w52, "IntegTime"=w60, "Stop Acq"=w61, "Accumulation"=w59, "ErrorIn(NoErr)"=w55, "Save"=w62, "AndorOpQ"=w65, "AndorAcqQ"=w64) -> ("error out"=w57:errorcluster, "Data out"=w53:i32[][])  [unwired: 2 out]
            n164 = local read "Save Bckgnd"() -> (w54:bool)
            n165 = case shown="Vrai" w54 {
              tunnel: w53 -> [_ w67]
              frame False {
              }
              frame True {
                n166 = Delete From Array(array=w67) -> (deleted portion=→"Background":i32[])  [unwired: 3 in, 1 out]
              }
            }
            n167 = flat-sequence {
              tunnel: [w71] -> w58
              tunnel: w57 -> [w71]
              frame #0 {
                n168 = local write "Aquiring"(FALSE) -> ()
              }
            }
          }
          frame "SetGain" {
            n169 = Variant To Data(error in=w74, type=0, Variant=w77) -> (data=w75:i32, error out=w73:errorcluster)
            n170 = call <userlib>:"SetPreAmpGain.vi"("error in (no error)"=w73, "index"=w75) -> ("error out"=w72:errorcluster)  [unwired: 1 out]
          }
          frame "AcquireLive" {
          }
          frame "SetInteg" {
            n171 = Variant To Data(type=u32 0, Variant=w86) -> (data=w85:u32)  [unwired: 1 in, 1 out]
            n172 = To Single Precision Float(number=w85) -> (single precision float=w88:sgl)
            n173 = local read "Accumulation"() -> (w83:u16)
            n174 = Divide(x=w88, y=sgl 1000.0) -> (x/y=w79:sgl)
            n175 = call <userlib>:"SetExposureTime.vi"("error in (no error)"=w81, "time"=w79) -> ("error out"=w80:errorcluster)  [unwired: 1 out]
            n176 = call <userlib>:"GetAcquisitionTimings.vi"("exposure input"=w79, "accumulate input"=w83, "error in (no error)"=w80) -> ("exposure"=w90:sgl, "accumulate"=→"accumulate":sgl, "error out"=w84:errorcluster)  [unwired: 8 in, 2 out]
            n177 = local write "AcqTime"(w90) -> ()
          }
        }
      }
      n178 = Release Queue(queue=w15, error in (no error)=w7) -> ()  [unwired: 1 in, 3 out]
    }
    frame Error {
    }
  }
  "error out" <- w5
  "AndorSpectro.lvclass Out" <- w3
